vi "ChildModuleTemplate.vi"(10 "SW Rev":T3={"AppName"="App Name", "Company"="Company Name", "Version"="0.0.1", "Date"="xx/xx/xx"}, 11 "Module Config":T1={"Name"="ModName", "Parent Q"=refnum, "Is Child?"=FALSE, "Index"=0, "Dirs"={"Root"=path "", "Config"=path "C:/ATE/Config", "Logs"=path "C:/ATE/Logs", "Reports"=path "C:/ATE/Reports", "App Data"=path "C:/ProgramData/MAIN"}}) -> ()   [LabVIEW 2016]
uses:
  <vilib>/KATE/Queues/Queue Utils.lvlib
  <vilib>/KATE/Module/Module Utils.lvlib
  <vilib>/KATE/Module/Public/Action - Window Tasks.ctl
  <vilib>/KATE/Event Log/Event Log.lvlib
  <vilib>/KATE/Module/Public/Error Report.ctl
  <vilib>/KATE/Scheduler/Scheduler.lvlib
  <vilib>/KATE/Files/File Utils.lvlib
  Utils/Config/Save Control States/Save Control - Action.ctl
  <vilib>/KATE/Queues/Q.Element.ctl
  <vilib>/KATE/Module/Module Config.ctl
  <vilib>/KATE/Module/Public/SW Version Info.ctl
  <vilib>/KATE/Module/Module.Working Dirs.ctl
panel:
  in  "Main UI Tab":enum32{"Operate", "Maint"}(tab)
  out "Simulate Indication":string="Simulating Instruments"
  out "Error":bool
  out "Title":string="Child Name"
  in  "Data Tab":enum32{"Operate", "Config"}(tab)
  in  "Control1":bool
  in  "Reset":bool
  in  "Maint":bool
  in  "Simulate En":bool
  in  "Exit":bool
  in  "Show Block Diagram":bool
  in  "Leave Maint":bool
  # "<Update Version and save as default values>"
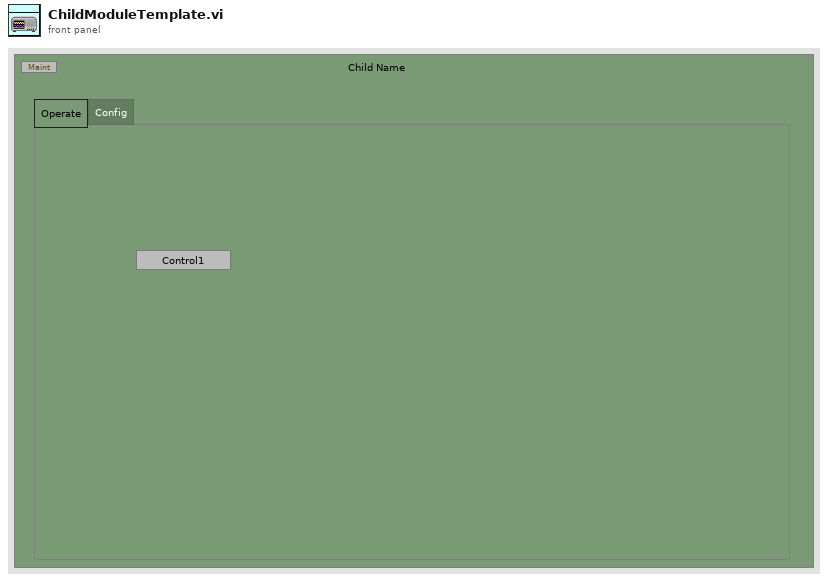
[diagram p1: front panel]
types:
  T1 = typedef "KATE_Lib.lvlib/Module Utils.lvlib/Module Config.ctl" = cluster{"Name":string, "Parent Q":refnum<queue>, "Is Child?":bool, "Index":i32, "Dirs":T2}
  T2 = typedef "KATE_Lib.lvlib/Module Utils.lvlib/Module.Working Dirs.ctl" = cluster{"Root":path, "Config":path, "Logs":path, "Reports":path, "App Data":path}
  T3 = typedef "KATE_Lib.lvlib/Module Utils.lvlib/SW Version Info.ctl" = cluster{"AppName":string, "Company":string, "Version":string, "Date":string}
  T4 = typedef "KATE_Lib.lvlib/Module Utils.lvlib/Module Sys Info.ctl" = cluster{"Main Q":refnum<queue>, "Exe":bool, "SW Rev":T5, "Self Ref":refnum<vi>, "Main Tab":refnum<vi>, "Pane":refnum<vi>, "Stop":cluster{"Ref":refnum<event-registration>, "Event":refnum<user-event>}, "Cfg":T1, "Services":cluster{"Name":string, "vi ref":refnum<vi>}[]}
  T5 = typedef "KATE_Lib.lvlib/Module Utils.lvlib/Module.SW Version Info.ctl" = cluster{"AppName":string, "Company":string, "Version":string, "Date":string}
  T6 = typedef "KATE_Lib.lvlib/Module Utils.lvlib/Action - Window Tasks.ctl" = enum16{"Resize()", "Show Panel(Bool)", "Show Scroll Bars(Bool)", "Dock to SubPanel(SubPanel Ref)", "Undock from SubPanel()", "Return to SubPanel()", "Go To Maint Tab()", "Show Maint Tab(Bool)", "Open Block Diagram()"}
  T7 = typedef "Save Control - Action.ctl" = enum16{"Read", "Save", "Add Single Ctrl", "Add Mult Ctrls", "Restore"}
  T8 = enum8{"Enabled", "Disabled", "Disabled and Grayed Out"}
  T9 = enum16{"Top Left", "Top Right", "Bottom Left", "Bottom Right"}
  T10 = typedef "KATE_Lib.lvlib/Module Utils.lvlib/Error Report.ctl" = cluster{"Cnt":i32, "Recent Error":errorcluster}
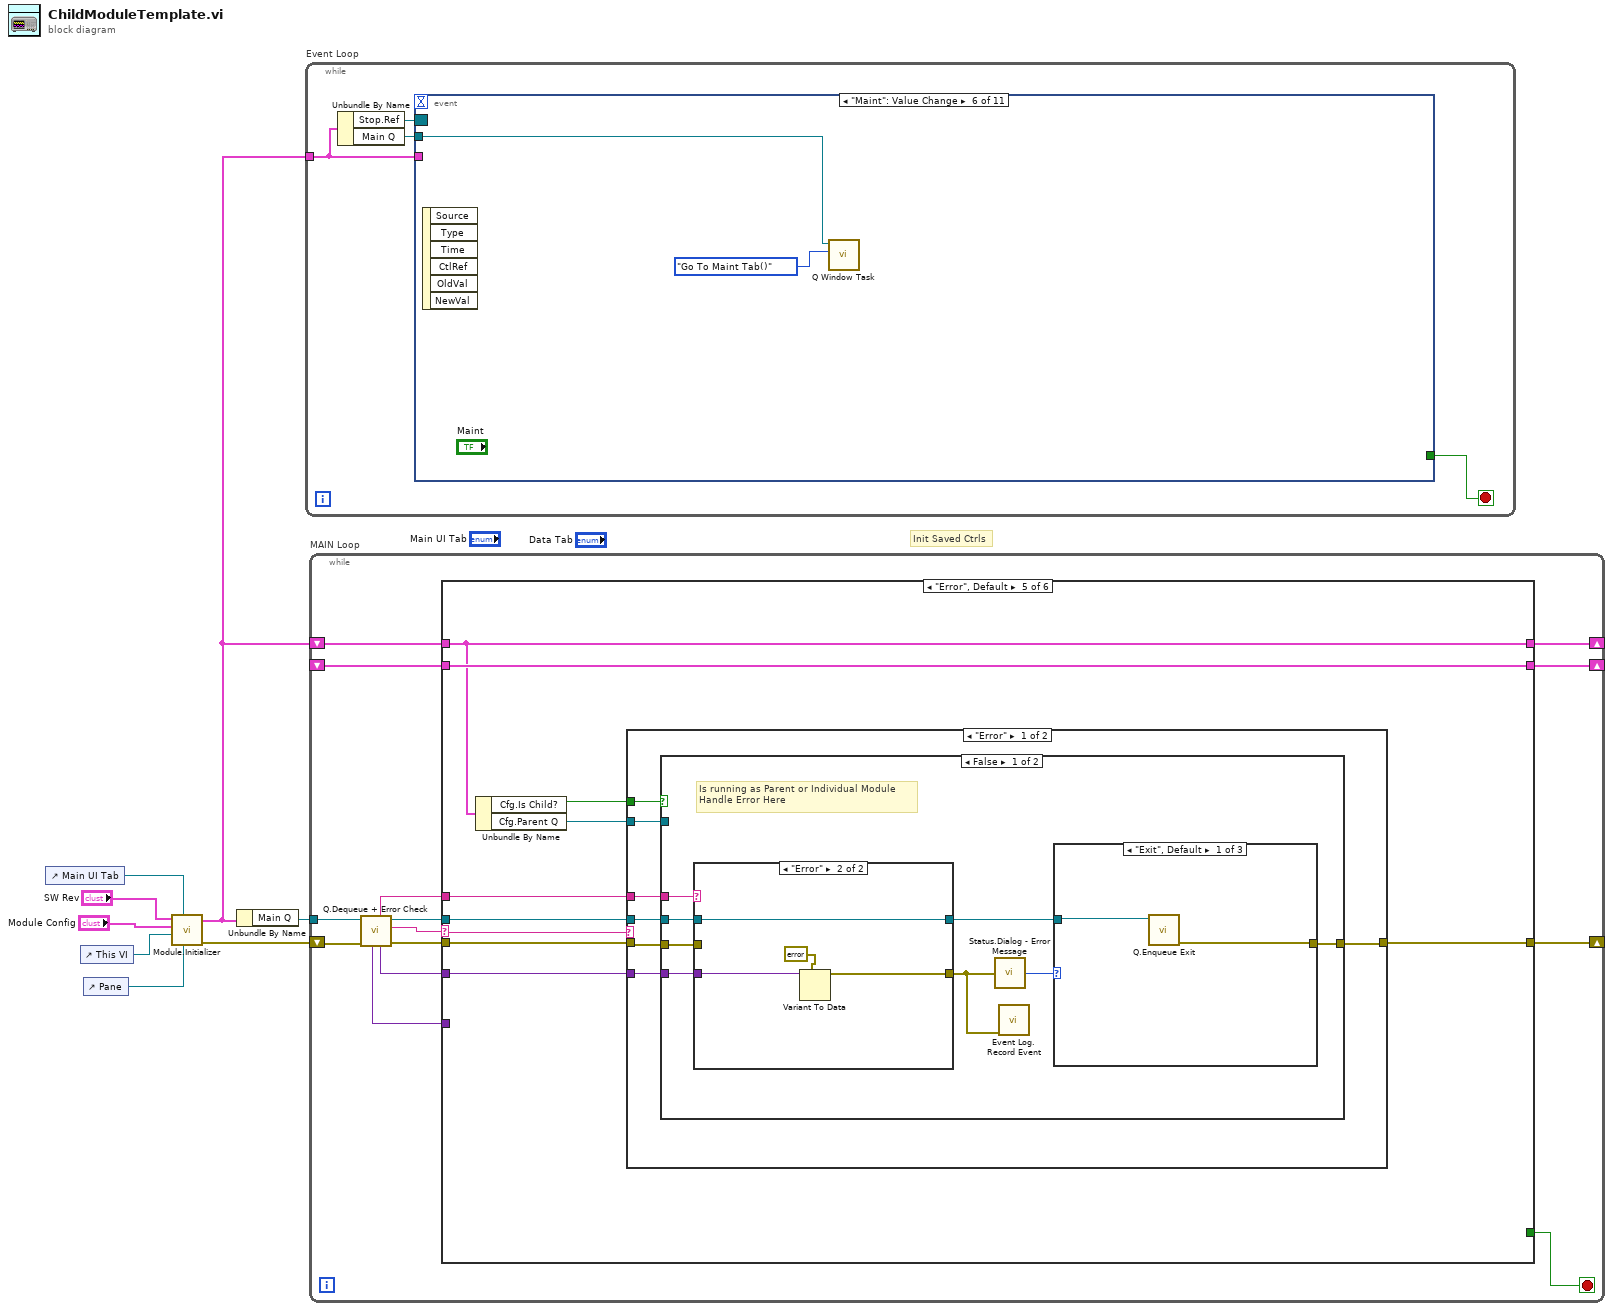
[diagram p0: block diagram]
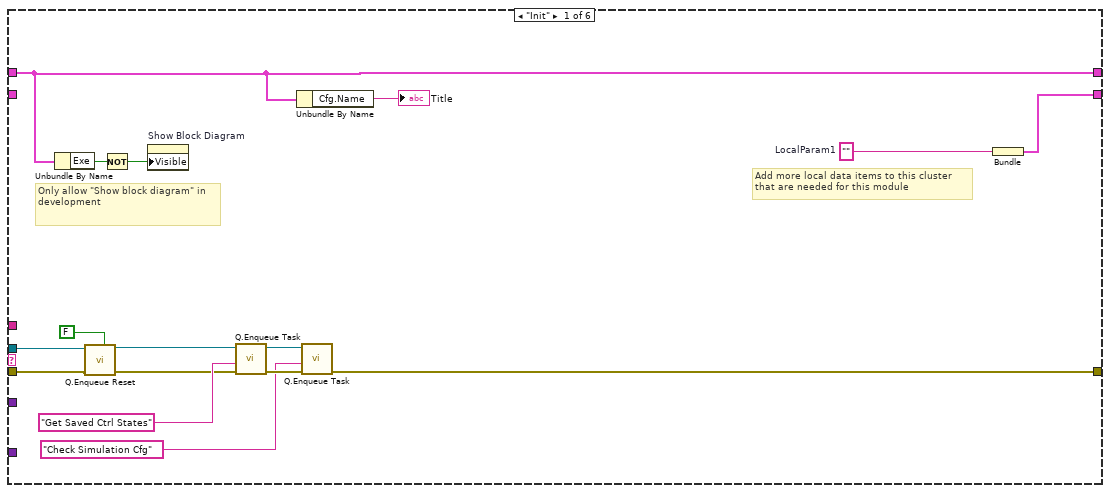
[diagram p2: hidden frame]
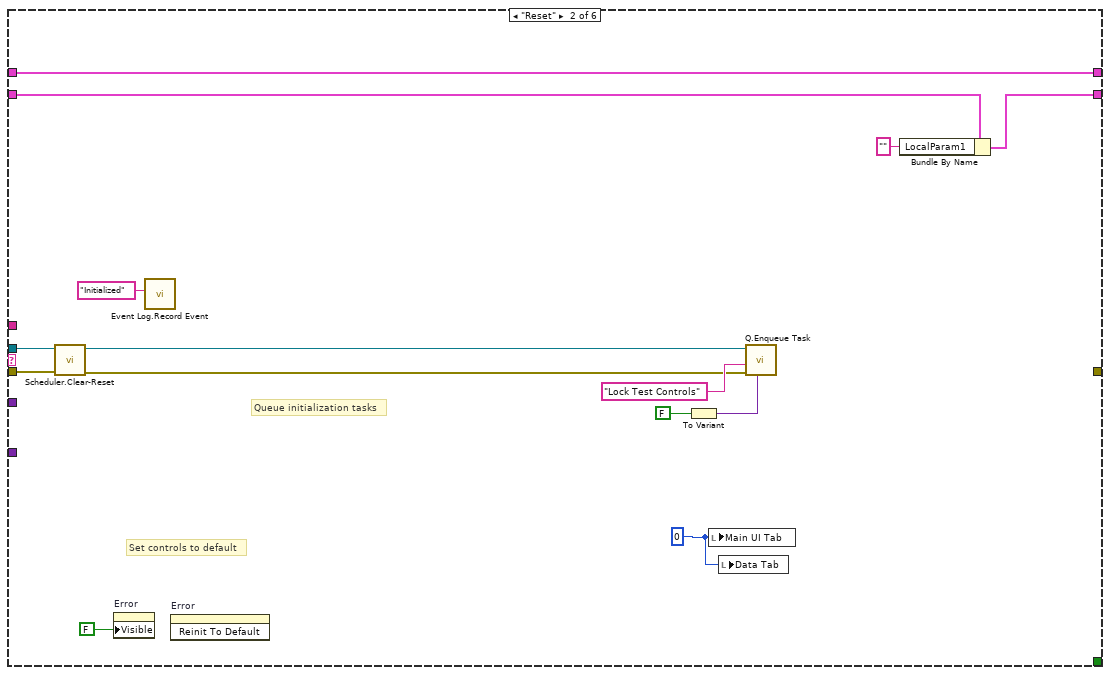
[diagram p3: hidden frame]
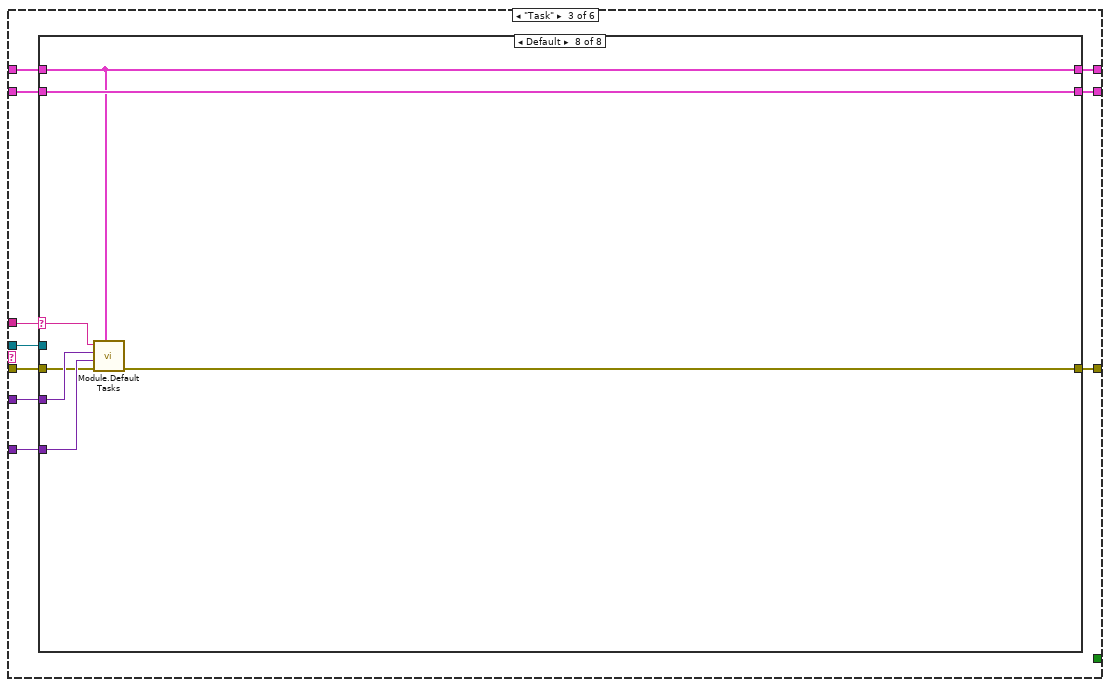
[diagram p4: hidden frame]
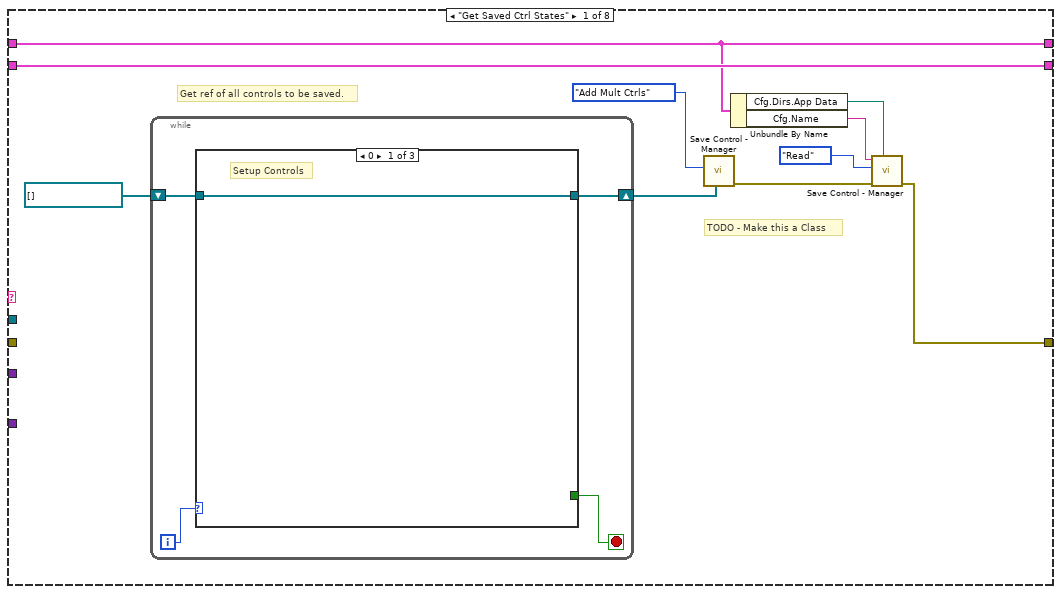
[diagram p5: hidden frame]
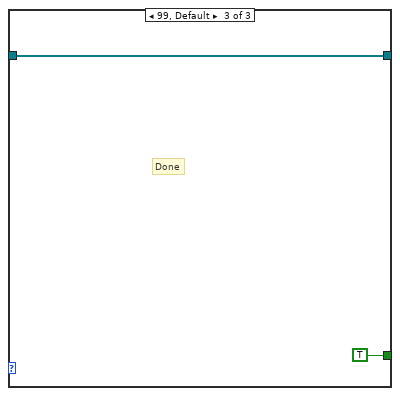
[diagram p7: hidden frame]
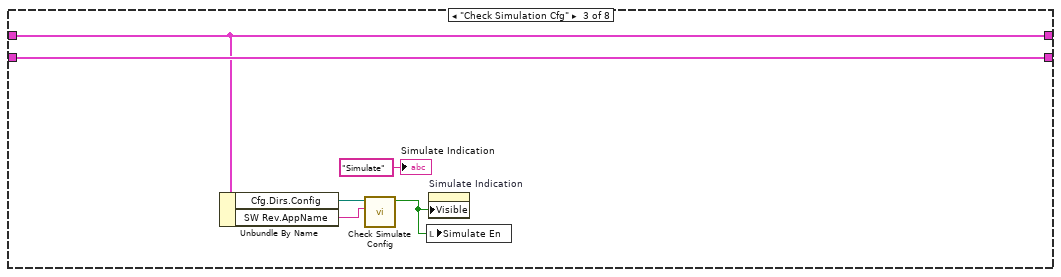
[diagram p9: hidden frame]
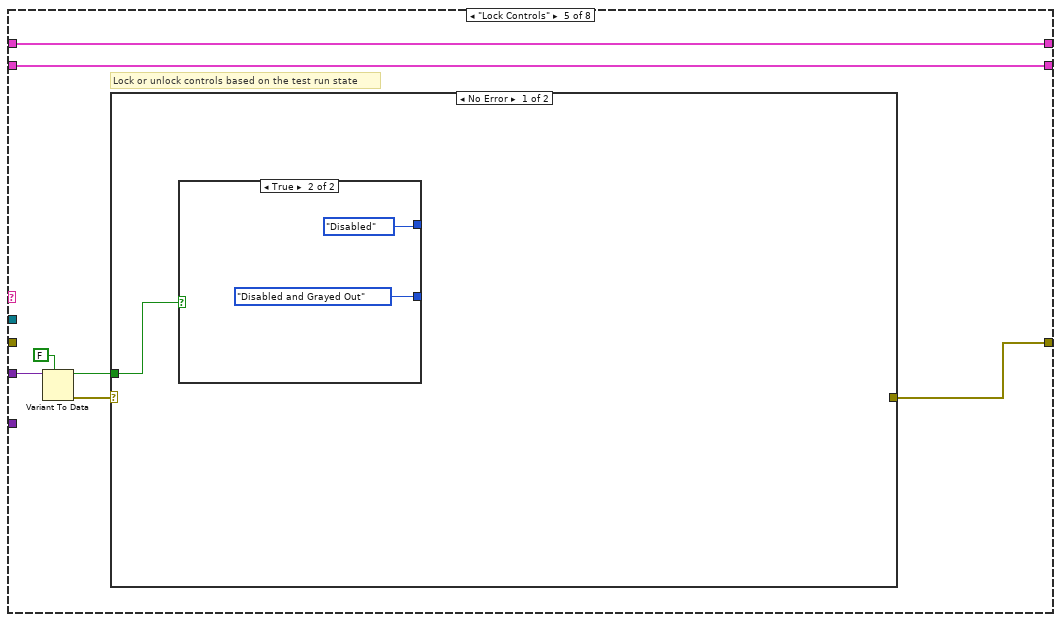
[diagram p11: hidden frame]
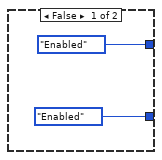
[diagram p12: hidden frame]
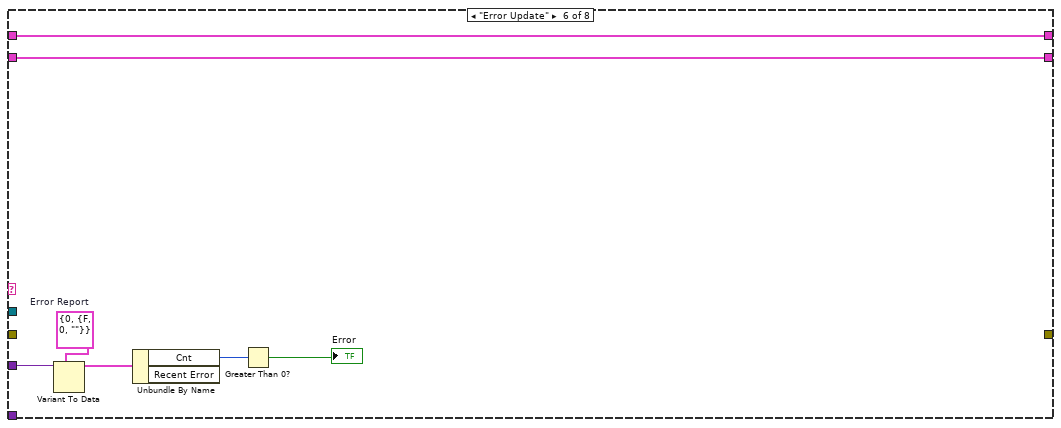
[diagram p14: hidden frame]
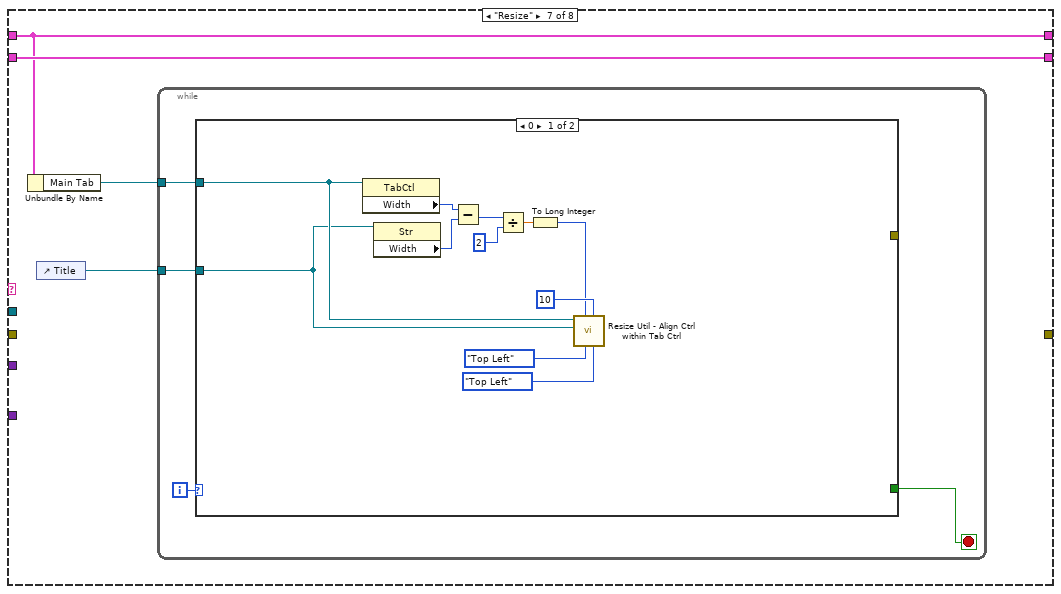
[diagram p15: hidden frame]
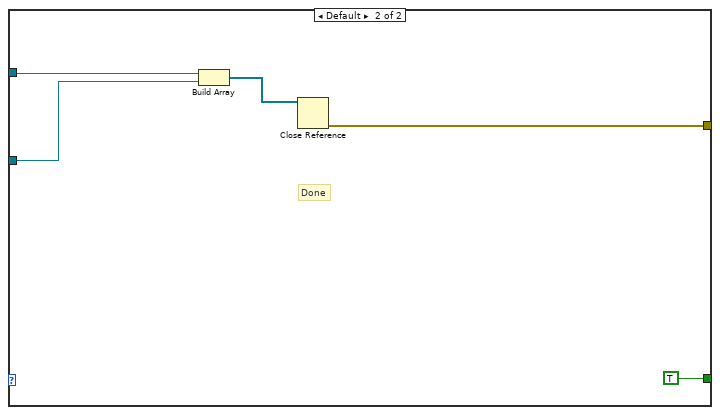
[diagram p16: hidden frame]
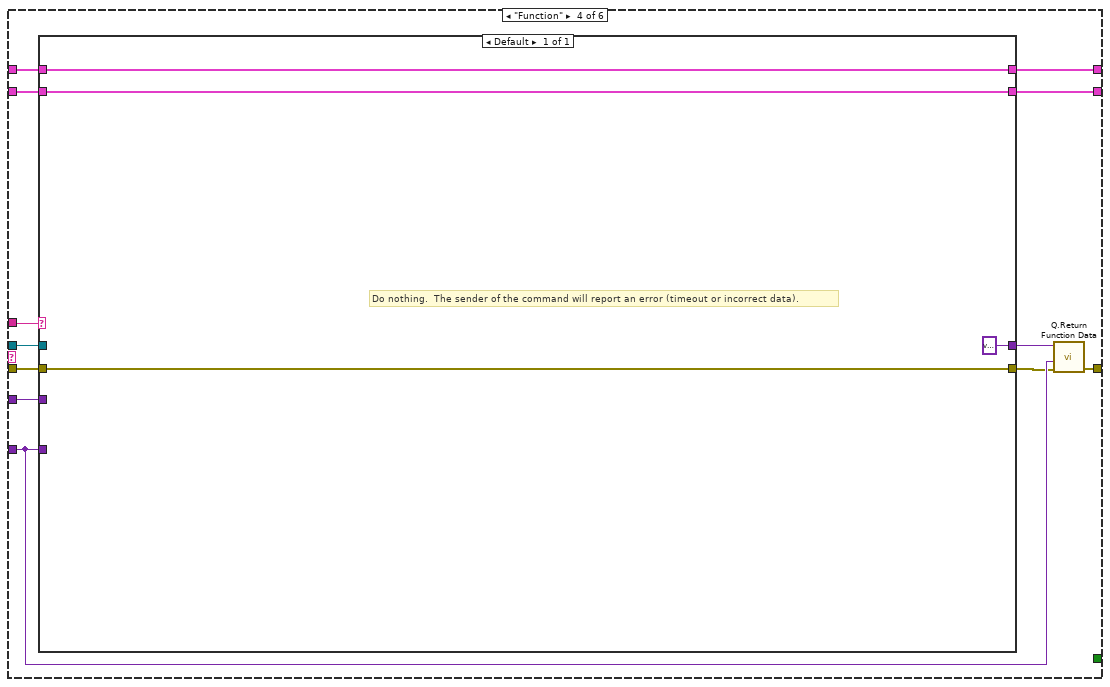
[diagram p17: hidden frame]
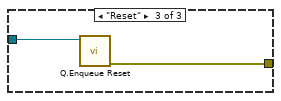
[diagram p19: hidden frame]
diagram:
  # "Init Saved Ctrls"
  n1 = control-ref of="Main UI Tab"() -> (w5:refnum<vi>)
  n2 = control-ref of="This VI"() -> (w4:refnum<vi>)
  n3 = control-ref of="Pane"() -> (w3:refnum<vi>)
  n4 = call <vilib>:"Module.Initializer.vi"("Pane"=w3, "Main Tab"=w5, "Self Ref"=w4, "Module Config"="Module Config", "SW Rev"="SW Rev") -> ("error out"=w8:errorcluster, "Sys"=w7:T4)  [unwired: 5 in]
  n5 = Unbundle By Name(w7) -> ("Main Q"=w6:refnum<queue>)
  n6 = while "Event Loop" {
    tunnel: w7 -> [w11]
    stop <- w12 stop-if-true
    n7 = Unbundle By Name(w11) -> ("Stop.Ref"=w10:refnum<event-registration>, "Main Q"=w9:refnum<queue>)
    n8 = event shown="[5] \"Maint\": Value Change" {
      selector: w10 -> [_ _ _ _ _ _ _ _ _ _ _]
      dyn-events: _ -> [_ _ _ _ _ _ _ _ _ _ _]
      timeout: _ -> [_ _ _ _ _ _ _ _ _ _ _]
      tunnel: [w16 TRUE _ _ _ _ _ w40 TRUE _ _] -> w12
      tunnel: w11 -> [w15 _ _ _ _ _ _ w38 _ w65 _]
      tunnel: w9 -> [w18 w28 w30 w32 w34 w36 _ w39 _ _ w67]
      event Panel Close? {
        n9 = event-data() -> ()  [unwired: 1 in, 4 out]
        n10 = Unbundle By Name(w15) -> ("Exe"=w13:bool, "Cfg.Is Child?"=w14:bool)
        n11 = case shown="False" w14 {
          tunnel: w18 -> [w22 w25]
          tunnel: [w20 TRUE] -> w17
          tunnel: [TRUE FALSE] -> w16
          tunnel: [_ w23] -> _
          tunnel: w13 -> [w19 _]
          frame False {
            # "Parent - Exit"
            n12 = call <vilib>:"Q.Enqueue Exit.vi"("Q In"=w22) -> ()  [unwired: 9 in, 2 out]
            n13 = Not(x=w19) -> (.not. x?=w20:bool)
          }
          frame True {
            # "Child - Hide Panel"
            n14 = call <vilib>:"Q Window Task.vi"("Action"=Action_-_Window_Tasks."Return to SubPanel()", "Q In"=w25) -> ("error out"=w23:errorcluster)  [unwired: 8 in, 1 out]
          }
        }
        n15 = event-data("Discard?"=w17) -> ()  [unwired: 1 in, 1 out]
      }
      event "Exit": Value Change {
        n16 = event-data() -> ()  [unwired: 1 in, 6 out]
        n17 = call <vilib>:"Q.Enqueue Exit.vi"("Q In"=w28) -> ()  [unwired: 9 in, 2 out]
      }
      event "Reset": Value Change {
        n18 = event-data() -> ()  [unwired: 1 in, 6 out]
        n19 = call <vilib>:"Q.Enqueue Reset.vi"("Q In"=w30) -> ()  [unwired: 9 in, 2 out]
      }
      event Panel Resize {
        n20 = event-data() -> ()  [unwired: 1 in, 8 out]
        n21 = call <vilib>:"Q Window Task.vi"("Action"=Action_-_Window_Tasks."Resize()", "Q In"=w32) -> ()  [unwired: 8 in, 2 out]
      }
      event "Show Block Diagram": Value Change {
        n22 = event-data() -> ()  [unwired: 1 in, 6 out]
        n23 = call <vilib>:"Q Window Task.vi"("Action"=Action_-_Window_Tasks."Open Block Diagram()", "Q In"=w34) -> ()  [unwired: 8 in, 2 out]
      }
      event "Maint": Value Change {
        n24 = event-data() -> ()  [unwired: 1 in, 6 out]
        n25 = call <vilib>:"Q Window Task.vi"("Action"=Action_-_Window_Tasks."Go To Maint Tab()", "Q In"=w36) -> ()  [unwired: 8 in, 2 out]
      }
      event "Leave Maint": Value Change {
        n26 = event-data() -> ()  [unwired: 1 in, 6 out]
        n27 = local write "Main UI Tab"(0) -> ()
      }
      event Menu Selection (User) {
        n28 = event-data() -> ("ItemTag"=w41:string)  [unwired: 1 in, 6 out]
        n29 = case shown="Default" w41 {
          tunnel: [_ TRUE _ _ _ _ _] -> w40
          tunnel: w39 -> [_ w42 _ w45 _ _ _]
          tunnel: [_ _ w44 _ w46 _ w51] -> _
          tunnel: w38 -> [_ _ _ _ w47 w50 w60]
          frame Default {
          }
          frame "Exit" {
            n30 = call <vilib>:"Q.Enqueue Exit.vi"("Q In"=w42) -> ()  [unwired: 9 in, 2 out]
          }
          frame "Show Event Log" {
            n31 = call <vilib>:"Event Log.Show.vi"() -> ("error out"=w44:errorcluster)  [unwired: 11 in]
          }
          frame "Reset" {
            n32 = call <vilib>:"Q.Enqueue Reset.vi"("Q In"=w45) -> ()  [unwired: 9 in, 2 out]
          }
          frame "Open Log Folder" {
            n33 = Unbundle By Name(w47) -> ("Cfg.Dirs.Logs"=w48:path)
            n34 = call <vilib>:"File.Open File or Folder.vi"("Path"=w48) -> ("Error Out"=w46:errorcluster)  [unwired: 10 in]
          }
          frame "Help.About" {
            n35 = Unbundle By Name(w50) -> ("SW Rev"=w49:T5)
            n36 = call "Help.About.vi"("SW Version"=w49) -> ()  [unwired: 11 in]
          }
          frame "Help.User Manual" {
            n37 = Unbundle By Name(w60) -> ("SW Rev.AppName"=w59:string)
            n38 = call <vilib>:"Application Directory.vi"() -> ("Application Directory"=w55:path)
            n39 = Build Path(base path=w55, name or relative path="Documentation") -> (appended path=w54:path)
            n40 = Concatenate Strings("User Manual, ", w59, ".pdf") -> (w53:string)
            n41 = Build Path(base path=w54, name or relative path=w53) -> (appended path=w52:path)
            n42 = call <vilib>:"File.Open File or Folder.vi"("Path"=w52) -> ("Error Out"=w51:errorcluster)  [unwired: 10 in]
          }
        }
      }
      event User Event {
        n43 = event-data() -> ()  [unwired: 1 in, 5 out]
      }
      event "Simulate En": Value Change {
        n44 = event-data() -> ()  [unwired: 1 in, 6 out]
        n45 = Unbundle By Name(w65) -> ("Cfg.Dirs.Config"=w64:path, "SW Rev.AppName"=w63:string)
        n46 = call "Save Simulate Config.vi"("Simulate"="Simulate En", "App Name"=w63, "Config Folder"=w64) -> ()  [unwired: 8 in, 1 out]
        n47 = property on="Simulate Indication" class="Str"("Visible"="Simulate En") -> ()  [unwired: 2 in, 2 out]
      }
      event "Control1": Value Change {
        # "This code is a template for how to handle a control event.  \nEnque one or more tasks to handle the control change event"
        n48 = event-data() -> ()  [unwired: 1 in, 6 out]
        n49 = To Variant(anything="Control1") -> (Variant=w68:variant)
        n50 = call <vilib>:"Q.Enqueue Task.vi"("Data1"=w68, "Task Name"="Control1", "Q In"=w67) -> ()  [unwired: 7 in, 2 out]
      }
    }
  }
  n51 = while "MAIN Loop" {
    shift-right: [w79] -> _
    shift-left: w8 -> [w77]
    shift-right: [w80] -> _
    shift-left: _ -> [w83]
    shift-right: [w81] -> _
    shift-left: w7 -> [w82]
    tunnel: w6 -> [w76]
    stop <- w70 stop-if-true
    n52 = call <vilib>:"Q.Dequeue + Error Check.vi"("Error In"=w77, "Q In"=w76) -> ("error out"=w78:errorcluster, "Cmd"=w75:string, "Q Out"=w74:refnum<queue>, "Data1"=w73:variant, "Sub"=w71:string, "Data2"=w72:variant)  [unwired: 4 in]
    n53 = case shown="\"Error\", Default" w75 {
      selector: w75 -> [_ _ _ _ w226 _]
      tunnel: w83 -> [_ w103 w122 w213 w228 w267]
      tunnel: w82 -> [w92 w107 w123 w214 w221 w269]
      tunnel: [w92 w107 w121 w212 w221 w269] -> w81
      tunnel: [w88 w109 w120 w211 w228 w267] -> w80
      tunnel: [w87 _ w114 w206 w227 w273] -> w79
      tunnel: w78 -> [w98 w112 w116 w207 w224 _]
      tunnel: w74 -> [w99 w113 w117 w208 w222 _]
      tunnel: w73 -> [_ _ w118 w209 w225 _]
      tunnel: w72 -> [_ _ w115 w205 _ _]
      tunnel: w71 -> [_ _ w119 w210 w223 _]
      tunnel: [_ _ _ _ _ TRUE] -> w70
      frame "Init" {
        w84 = ""  # LocalParam1
        # "Add more local data items to this cluster \nthat are needed for this module"
        # "Only allow \"Show block diagram\" in development"
        n54 = Unbundle By Name(w92) -> ("Exe"=w96:bool)
        n55 = call <vilib>:"Q.Enqueue Reset.vi"("Top of Q(T)"=FALSE ("Flush Q"), "Error In"=w98, "Q In"=w99) -> ("error out"=w85:errorcluster, "Q Out"=w86:refnum<queue>)  [unwired: 7 in]
        n56 = Not(x=w96) -> (.not. x?=w95:bool)
        n57 = property on="Show Block Diagram" class="Bool"("Visible"=w95) -> ()  [unwired: 2 in, 2 out]
        n58 = call <vilib>:"Q.Enqueue Task.vi"("Error In"=w85, "Task Name"="Get Saved Ctrl States", "Q In"=w86) -> ("error out"=w90:errorcluster, "Q Out"=w91:refnum<queue>)  [unwired: 7 in]
        n59 = Unbundle By Name(w92) -> ("Cfg.Name"=→"Title":string)
        n60 = call <vilib>:"Q.Enqueue Task.vi"("Error In"=w90, "Task Name"="Check Simulation Cfg", "Q In"=w91) -> ("error out"=w87:errorcluster)  [unwired: 7 in, 1 out]
        n61 = Bundle("LocalParam1"=w84) -> (w88:cluster{"LocalParam1":string})  [unwired: 1 in]
      }
      frame "Reset" {
        w110 = 0
        # "Set controls to default"
        # "Queue initialization tasks"
        n62 = call <vilib>:"Scheduler.Clear-Reset.vi"("error in"=w112, "Q In"=w113) -> ("error out"=w102:errorcluster, "Q Out"=w101:refnum<queue>)  [unwired: 8 in]
        n63 = property on="Error" class="Bool (strict)"("Visible"=FALSE) -> ()  [unwired: 2 in, 2 out]
        n64 = call <vilib>:"Event Log.Record Event.vi"("Message"="Initialized") -> ()  [unwired: 10 in, 1 out]
        n65 = invoke on="Error" class="Bool (strict)" method="Reinit To Default"() -> ()  [unwired: 3 in, 3 out]
        n66 = To Variant(anything=FALSE) -> (Variant=w105:variant)
        n67 = local write "Main UI Tab"(w110) -> ()
        n68 = local write "Data Tab"(w110) -> ()
        n69 = call <vilib>:"Q.Enqueue Task.vi"("Data1"=w105, "Error In"=w102, "Task Name"="Lock Test Controls", "Q In"=w101) -> ()  [unwired: 6 in, 2 out]
        n70 = Bundle By Name(cluster=w103, "LocalParam1"="") -> (w109:cluster{"LocalParam1":string})
      }
      frame "Task" {
        n71 = case shown="Default" w119 {
          selector: w119 -> [_ _ _ _ _ _ _ w200]
          tunnel: w123 -> [w126 w143 w144 w151 w158 w171 w174 w201]
          tunnel: w122 -> [w133 w142 w149 w150 w157 w170 w175 w202]
          tunnel: [w126 w143 w144 w151 w158 w171 w174 w201] -> w121
          tunnel: [w133 w142 w149 w150 w157 w170 w175 w202] -> w120
          tunnel: w118 -> [_ _ _ _ w156 w169 _ w199]
          tunnel: w117 -> [_ _ _ _ _ _ _ _]
          tunnel: w116 -> [_ _ _ _ _ _ _ w197]
          tunnel: w115 -> [_ _ _ _ _ _ _ w198]
          tunnel: [w124 _ _ _ w152 _ _ w196] -> w114
          frame "Get Saved Ctrl States" {
            # "TODO - Make this a Class"
            # "Get ref of all controls to be saved."
            n72 = while {
              shift-right: [w135] -> w130
              shift-left: refnum<vi>[] [] -> [w136]
              i -> [w137]
              stop <- w134 stop-if-true
              n73 = case shown="0" w137 {
                tunnel: w136 -> [w138 w139 w141]
                tunnel: [w138 w139 w141] -> w135
                tunnel: [_ _ TRUE] -> w134
                frame 0 {
                  # "Setup Controls"
                }
                frame 1 {
                  # "Main Controls"
                }
                frame 99, Default {
                  # "Done"
                }
              }
            }
            n74 = call "Save Control - Manager.vi"("Ctrl Array"=w130, "Action"=Save_Control_-_Action."Add Mult Ctrls") -> ("error out"=w125:errorcluster)  [unwired: 9 in]
            n75 = Unbundle By Name(w126) -> ("Cfg.Dirs.App Data"=w127:path, "Cfg.Name"=w128:string)
            n76 = call "Save Control - Manager.vi"("App Data Dir"=w127, "error in"=w125, "Action"=Save_Control_-_Action."Read", "App Name"=w128) -> ("error out"=w124:errorcluster)  [unwired: 7 in]
          }
          frame "Control1" {
            # "Handle Control state change"
          }
          frame "Check Simulation Cfg" {
            n77 = Unbundle By Name(w144) -> ("Cfg.Dirs.Config"=w148:path, "SW Rev.AppName"=w147:string)
            n78 = call "Check Simulate Config.vi"("App Name"=w147, "Config Folder"=w148) -> ("Simulate"=w145:bool)  [unwired: 9 in]
            n79 = local write "Simulate En"(w145) -> ()
            n80 = property on="Simulate Indication" class="Str"("Visible"=w145) -> ()  [unwired: 2 in, 2 out]
            "Simulate Indication" <- "Simulate" ("Simulate Indication")
          }
          frame "Initialization Done" {
          }
          frame "Lock Controls" {
            # "Lock or unlock controls based on the test run state"
            n81 = Variant To Data(type=FALSE, Variant=w156) -> (data=w153:bool, error out=w154:errorcluster)  [unwired: 1 in]
            n82 = case shown="No Error" w154 {
              selector: w154 -> [_ w164]
              tunnel: w153 -> [w159 _]
              tunnel: [_ w164] -> w152
              frame No Error {
                n83 = case shown="True" w159 {
                  tunnel: [T8."Enabled" ("Disabled") T8."Disabled and Grayed Out" ("Disabled")] -> _
                  tunnel: [T8."Enabled" ("Disabled") T8."Disabled" ("Disabled")] -> _
                  frame False {
                  }
                  frame True {
                  }
                }
              }
              frame Error {
              }
            }
          }
          frame "Error Update" {
            w168 = T10 {"Cnt"=0, "Recent Error"={"status"=FALSE, "code"=0, "source"=""}}  # Error Report
            n84 = Variant To Data(type=w168, Variant=w169) -> (data=w167:T10)  [unwired: 1 in, 1 out]
            n85 = Unbundle By Name(w167) -> ("Cnt"=w166:i32)  [unwired: 1 out]
            n86 = Greater Than 0?(x=w166) -> (x > 0?=→"Error":bool)
          }
          frame "Resize" {
            n87 = Unbundle By Name(w174) -> ("Main Tab"=w173:refnum<vi>)
            n88 = control-ref of="Title"() -> (w172:refnum<vi>)
            n89 = while {
              tunnel: w173 -> [w177]
              tunnel: w172 -> [w176]
              i -> [w179]
              stop <- w178 stop-if-true
              n90 = case shown="0" w179 {
                tunnel: [_ TRUE] -> w178
                tunnel: w177 -> [w188 w194]
                tunnel: w176 -> [w180 w193]
                tunnel: [_ w191] -> _
                frame 0 {
                  n91 = property class="TabCtl"(reference=w188) -> ("Width"=w185:u32)  [unwired: 1 in, 2 out]
                  n92 = property class="Str"(reference=w180) -> ("Width"=w184:u32)  [unwired: 1 in, 2 out]
                  n93 = Subtract(x=w185, y=w184) -> (x-y=w183:u32)
                  n94 = Divide(x=w183, y=2) -> (x/y=w182:dbl)
                  n95 = To Long Integer(number=w182) -> (32bit integer=w181:i32)
                  n96 = call <vilib>:"Resize Util - Align Ctrl within Tab Ctrl.vi"("Child Ref Pos"=T9."Top Left", "dY"=10 ("dX"), "Parent Ref Pos"=T9."Top Left", "dX"=w181, "Child Ctrl"=w180, "Parent Tab Ctrl"=w188) -> ()  [unwired: 3 in, 3 out]
                }
                frame Default {
                  # "Done"
                  n97 = Build Array(w194, w193) -> (w192:refnum<vi>[])
                  n98 = Close Reference(reference=w192) -> (error out=w191:errorcluster)  [unwired: 1 in]
                }
              }
            }
          }
          frame Default {
            n99 = call <vilib>:"Module.Default Tasks.vi"("Sys"=w201, "error in"=w197, "Data2"=w198, "Data1"=w199, "Sub"=w200) -> ("error out"=w196:errorcluster)  [unwired: 6 in]
          }
        }
      }
      frame "Function" {
        n100 = case shown="Default" w210 {
          tunnel: w214 -> [w217]
          tunnel: w213 -> [w218]
          tunnel: [w217] -> w212
          tunnel: [w218] -> w211
          tunnel: w209 -> [_]
          tunnel: w208 -> [_]
          tunnel: w207 -> [w215]
          tunnel: w205 -> [_]
          tunnel: [w215] -> w204
          tunnel: [variant] -> w203
          frame Default {
            # "Do nothing.  The sender of the command will report an error (timeout or incorrect data)."
          }
        }
        n101 = call <vilib>:"Q.Return Function Data.vi"("error in"=w204, "Data2"=w205, "Ret Data"=w203) -> ("error out"=w206:errorcluster)  [unwired: 8 in]
      }
      frame "Error", Default {
        n102 = Unbundle By Name(w221) -> ("Cfg.Is Child?"=w220:bool, "Cfg.Parent Q"=w219:refnum<queue>)
        n103 = case shown="\"Error\"" w226 {
          selector: w226 -> [_ w260]
          tunnel: [w231 w261] -> w227
          tunnel: w225 -> [w235 _]
          tunnel: w224 -> [w233 _]
          tunnel: w223 -> [w234 _]
          tunnel: w222 -> [w232 _]
          tunnel: w220 -> [w230 _]
          tunnel: w219 -> [w229 _]
          frame "Error" {
            n104 = case shown="False" w230 {
              tunnel: w235 -> [w243 _]
              tunnel: w234 -> [w242 _]
              tunnel: w233 -> [w241 w256]
              tunnel: w232 -> [w239 _]
              tunnel: [w237 w254] -> w231
              tunnel: w229 -> [_ w259]
              frame False {
                # "Is running as Parent or Individual Module\nHandle Error Here"
                n105 = case shown="\"Error\"" w242 {
                  tunnel: w243 -> [_ w253]
                  tunnel: w241 -> [w249 _]
                  tunnel: [w249 w251] -> w236
                  tunnel: w239 -> [w248 w250]
                  tunnel: [w248 w250] -> w238
                  frame Default {
                  }
                  frame "Error" {
                    n106 = Variant To Data(type=errorcluster {"status"=FALSE, "code"=0, "source"=""} ("error constant"), Variant=w253) -> (data=w251:errorcluster)  [unwired: 1 in, 1 out]
                  }
                }
                n107 = call <vilib>:"Status.Dialog - Error Message.vi"("error in"=w236) -> ("Selection"=w240:enum16{"Exit", "Reset", "Ignore"})
                n108 = call <vilib>:"Event Log.Record Event.vi"("error in"=w236) -> ()  [unwired: 10 in, 1 out]
                n109 = case shown="\"Exit\", Default" w240 {
                  tunnel: w238 -> [w245 _ w247]
                  tunnel: [w244 _ w246] -> w237
                  frame "Exit", Default {
                    n110 = call <vilib>:"Q.Enqueue Exit.vi"("Q In"=w245) -> ("error out"=w244:errorcluster)  [unwired: 9 in, 1 out]
                  }
                  frame "Ignore" {
                  }
                  frame "Reset" {
                    n111 = call <vilib>:"Q.Enqueue Reset.vi"("Q In"=w247) -> ("error out"=w246:errorcluster)  [unwired: 9 in, 1 out]
                  }
                }
              }
              frame True {
                w257 = "Error" ("Cmd")
                # "Is a child.  Pass the error to the Parent Module"
                n112 = To Variant(anything=w256) -> (Variant=w255:variant)
                n113 = call <vilib>:"Q.Enqueue Item.vi"("Top of Q"=TRUE, "Data1"=w255, "Sub"=w257, "Cmd"=w257, "Q In"=w259) -> ("error out"=w254:errorcluster)  [unwired: 5 in, 1 out]
              }
            }
          }
          frame Default {
            n114 = Concatenate Strings("Undefined State: \"", w260, "\".") -> (w262:string)
            n115 = Bundle By Name(cluster=errorcluster {"status"=TRUE, "code"=-5000, "source"=""} ("error constant"), "source"=w262) -> (w261:errorcluster)
          }
        }
      }
      frame "Exit" {
        # "Save control states"
        n116 = Unbundle By Name(w269) -> ("Cfg.Dirs.App Data"=w266:path, "Cfg.Name"=w270:string)
        n117 = call "Save Control - Manager.vi"("App Data Dir"=w266, "Action"=Save_Control_-_Action."Save", "App Name"=w270) -> ("error out"=w268:errorcluster)  [unwired: 8 in]
        n118 = call <vilib>:"Clear Errors.vi"("error in (no error)"=w268) -> ()  [unwired: 5 in, 2 out]
        n119 = call <vilib>:"Module.Destructor.vi"("Sys"=w269) -> ("error out"=w273:errorcluster)  [unwired: 10 in]
      }
    }
  }
